vi "addArgument_NumpyArray_Int32.vi"(7 "argument name":string, 8 "error in (no error)":errorcluster, 9 "argument list in":T1[](array[typedef]), 10 "data":i32[](array[numeric]), 11 "LabVIEW-Python-Interface in":refnum<class "PyLVi.lvclass">) -> (0 "error out":errorcluster, 1 "argument list out":T1[](array[typedef]), 3 "LabVIEW-Python-Interface out":refnum<class "PyLVi.lvclass">)   [LabVIEW 2016, in "PyLVi.lvlib" / "PyLVi.lvclass"]
uses:
  PyLVi.lvclass
  Controls/ArgumentStructure.ctl
  Controls/DescriptorStructure.ctl
  Controls/ArgumentType.ctl
  Controls/DataType.ctl
panel:
  out "data string":string
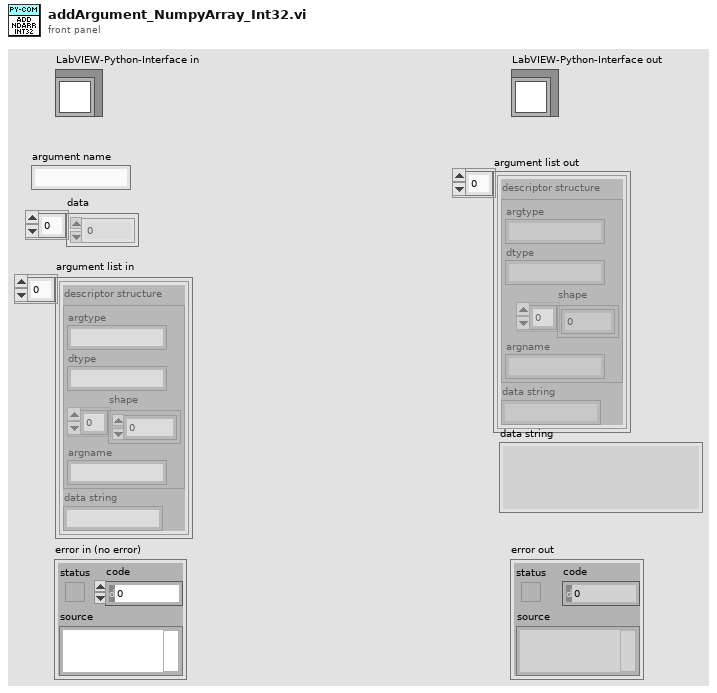
[diagram p1: front panel]
types:
  T1 = typedef "PyLVi.lvlib/PyLVi.lvclass/ArgumentStructure.ctl" = cluster{"descriptor structure":T2, "data string":string}
  T2 = typedef "PyLVi.lvlib/PyLVi.lvclass/DescriptorStructure.ctl" = cluster{"argtype":string, "dtype":string, "shape":u32[], "argname":string}
  T3 = enum16{"big-endian, network order", "native, host order", "little-endian"}
  T4 = typedef "PyLVi.lvlib/PyLVi.lvclass/DataType.ctl" = enum16{"bool", "string", "int16", "int32", "float32", "float64", "complex128"}
  T5 = typedef "PyLVi.lvlib/PyLVi.lvclass/ArgumentType.ctl" = enum8{"bool", "numeric", "string", "dict", "ndarray", "ndarray2d"}
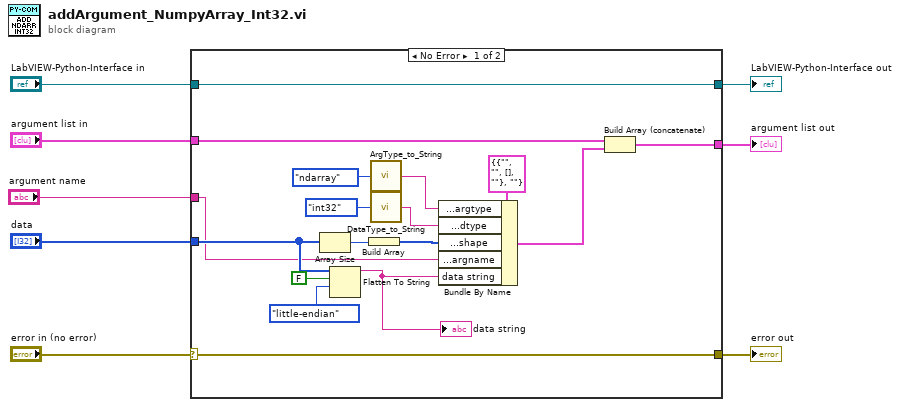
[diagram p0: block diagram]
diagram:
  n1 = case shown="No Error" "error in (no error)" {
    selector: "error in (no error)" -> [w25 w27]
    tunnel: [w25 w27] -> w7
    tunnel: [w24 w28] -> w5
    tunnel: "LabVIEW-Python-Interface in" -> [w24 w28]
    tunnel: "data" -> [w15 _]
    tunnel: "argument list in" -> [w20 w26]
    tunnel: [w18 w26] -> w2
    tunnel: "argument name" -> [w9 _]
    frame No Error {
      n2 = Array Size(array=w15) -> (size(s)=w22:i32)
      n3 = Flatten To String(anything=w15, prepend array or string size? (T)=FALSE, byte order (0:big-endian, network order)=T3."little-endian") -> (data string=w14:string)  [unwired: 1 in, 2 out]
      "data string" <- w14
      n4 = Build Array(w22) -> (w21:i32[])
      n5 = call "ArgType_to_String.vi"("arg type"=ArgumentType."ndarray" ("descriptor structure.argtype")) -> ("arg type string"=w11:string)  [unwired: 4 in]
      n6 = call "DataType_to_String.vi"("data type"=DataType."int32" ("descriptor structure.dtype")) -> ("data type string"=w10:string)  [unwired: 4 in]
      n7 = Bundle By Name(cluster=T1 {"descriptor structure"={"argtype"="", "dtype"="", "shape"=[], "argname"=""}, "data string"=""} ("argument structure"), "descriptor structure.argtype"=w11, "descriptor structure.dtype"=w10, "descriptor structure.shape"=w21, "descriptor structure.argname"=w9, "data string"=w14) -> (w19:T1)
      n8 = Build Array (concatenate)(w20, w19) -> (w18:T1[])
    }
    frame Error {
    }
  }
  "error out" <- w7
  "LabVIEW-Python-Interface out" <- w5
  "argument list out" <- w2
